vi "ORS_Fit_Recalibration_Fringes_Jay.vi"(0 "polynomial order":i32=2, 1 "n Recalibration Fringes":dbl[][](array[numeric]), 5 "polynomial fit algorithm":T1(ring), 7 "moving average half width":i32=1, 9 "interpolation method":i32(ring)=2 items=["nearest", "linear", "spline", "cubic Hermite", "Lagrange"], 11 "doPolyFit":bool, 12 "Offset":i32, 14 "Length":i32) -> (4 "maxphase":dbl, 6 "phase":dbl[](array[numeric]) format="%0.2f", 10 "inverted phase":dbl[](array[numeric]) format="%0.2f", 15 "rel.phase error":dbl[](array[numeric]) format="%0.2f")   [LabVIEW 2024]
uses:
  <vilib>/Analysis/baseanly.llb/Mean (DBL).vi
  <vilib>/Analysis/3filter.llb/Zero Phase Filter (DBL).vi
  <vilib>/Analysis/NI_AALPro.lvlib
  <vilib>/ptbypt/NI_PtbyPt.lvlib
  <vilib>/Analysis/NI_AALBase.lvlib
panel:
  out "CaliBackgroud":dbl[](graph)
  out "size(s)":i32[](array[numeric])
  out "Input":dbl[][](graph)
  out "Waveform Graph":dbl[](graph)
  out "element":dbl
  out "Mean fringes":dbl[][](graph)
  out "Unwrapped Hilbert phase":dbl[][](graph)
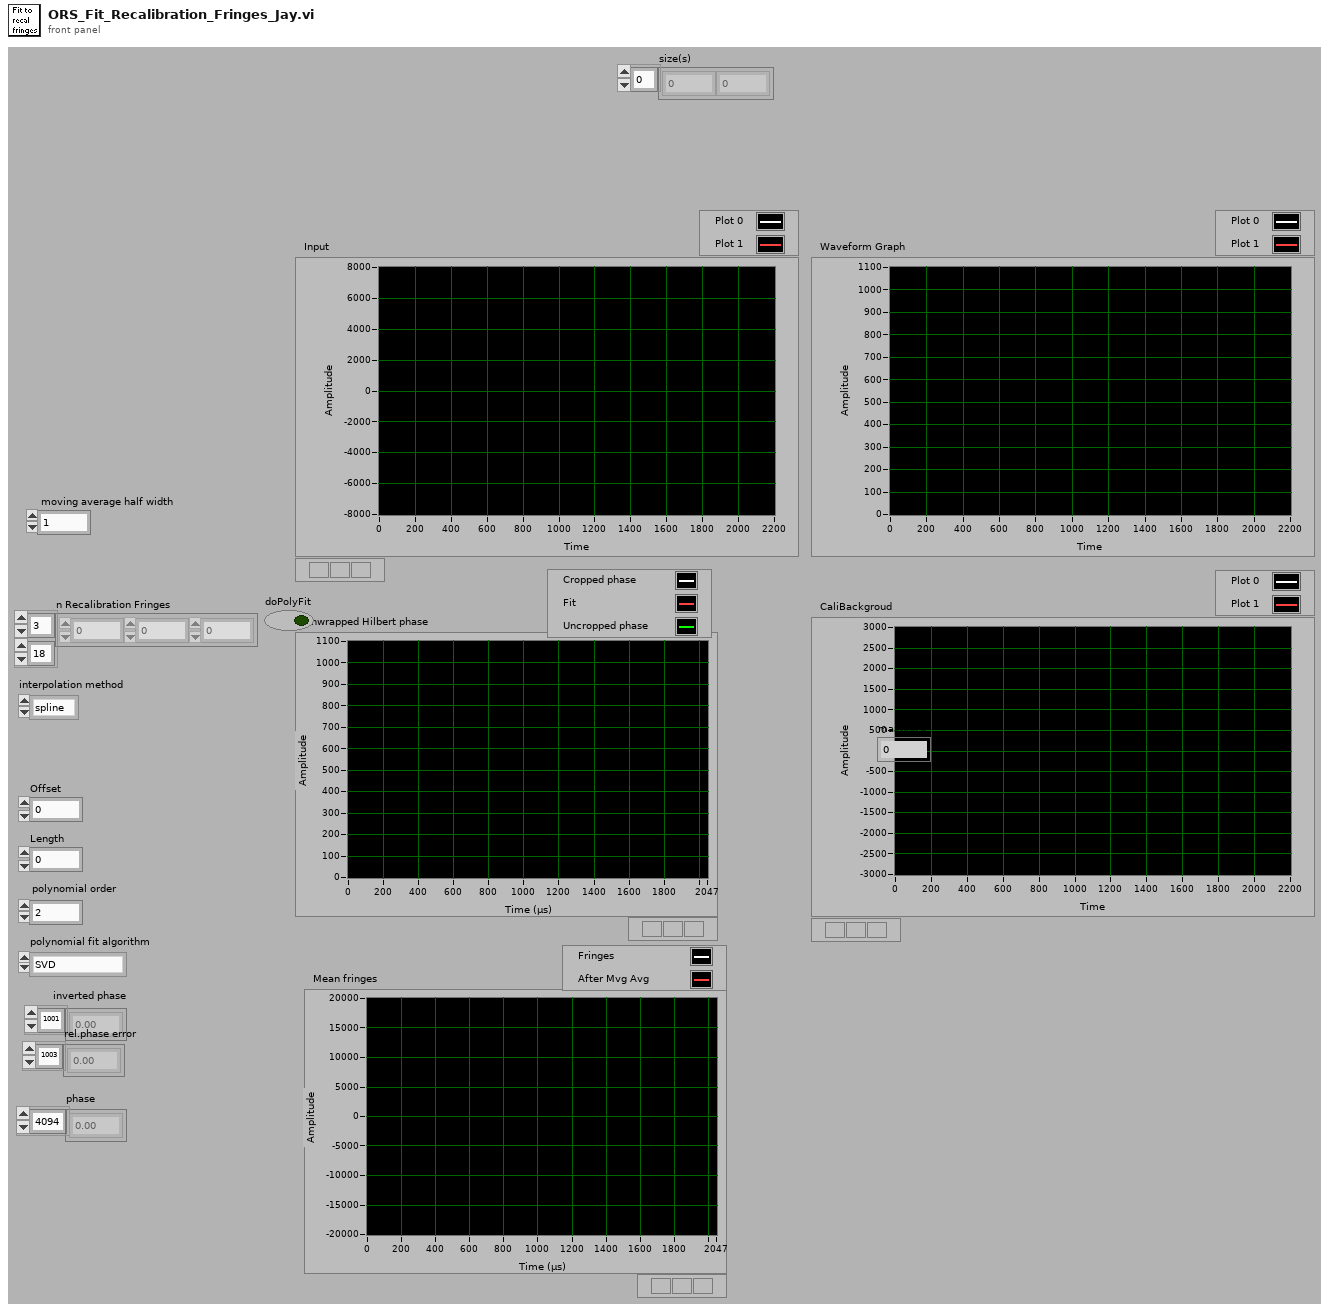
[diagram p1: front panel]
types:
  T1 = enum32{"SVD", "Givens", "Givens2", "Householder", "LU Decomposition", "Cholesky"}
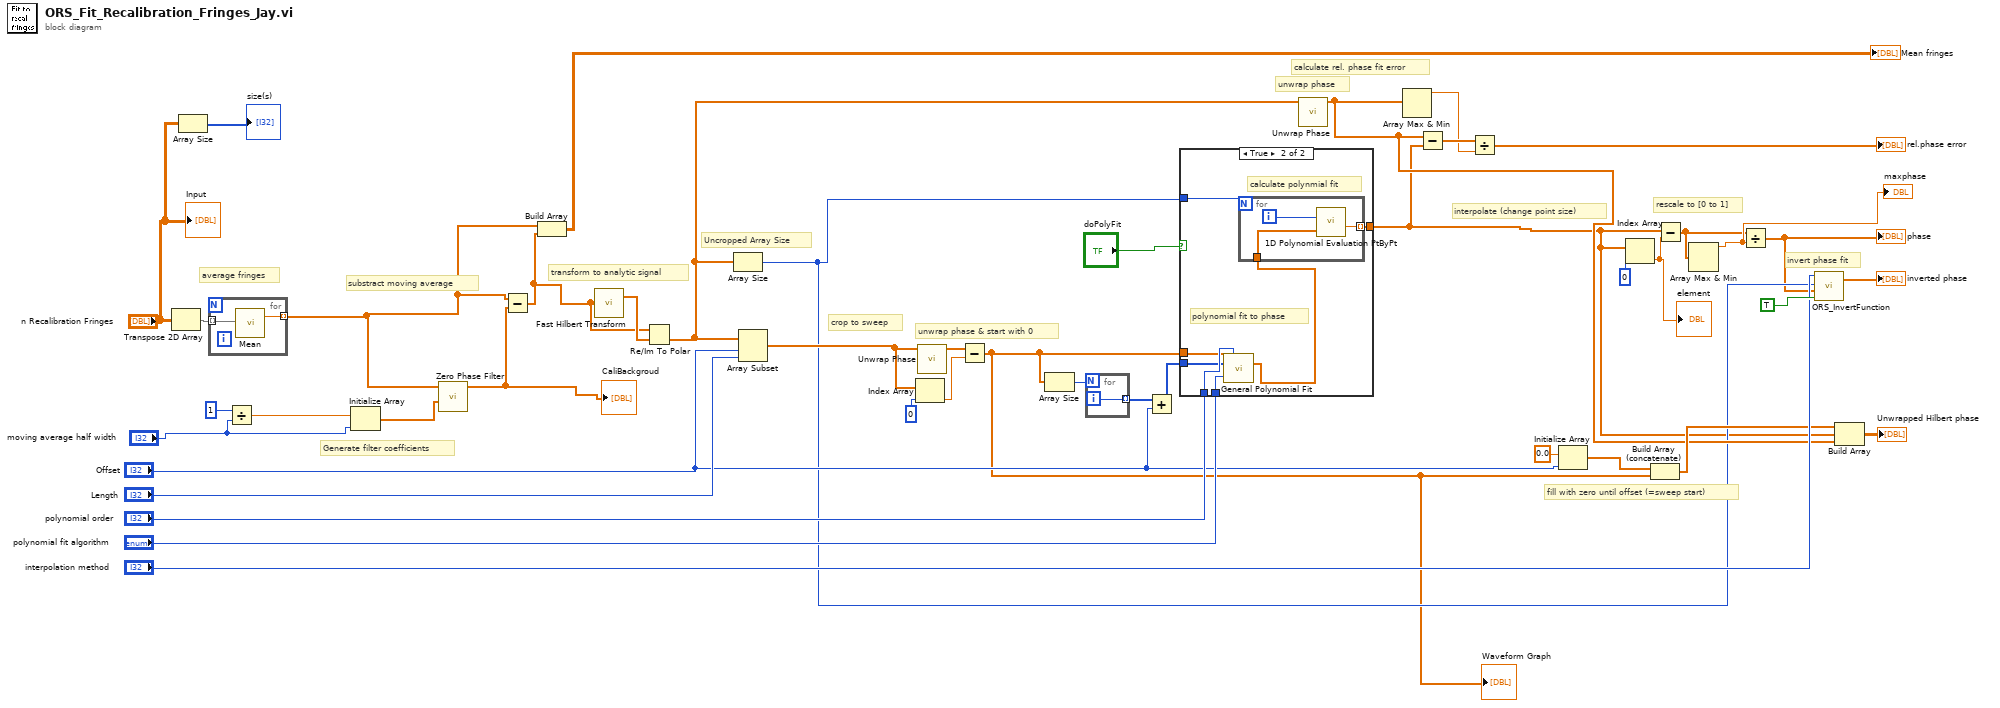
[diagram p0: block diagram]
diagram:
  # "Generate filter coefficients"
  # "transform to analytic signal"
  # "unwrap phase"
  # "average fringes"
  # "fill with zero until offset (=sweep start)"
  # "unwrap phase & start with 0"
  # "Uncropped Array Size"
  # "calculate rel. phase fit error"
  # "rescale to [0 to 1]"
  # "interpolate (change point size)"
  # "substract moving average"
  # "invert phase fit"
  # "crop to sweep"
  n1 = Transpose 2D Array(2D array="n Recalibration Fringes") -> (transposed array=w11:dbl[][])
  n2 = Array Size(array="n Recalibration Fringes") -> (size(s)=→"size(s)":i32[])
  n3 = for {
    tunnel: w11 -> [w46] mode=indexing
    tunnel: [w45] -> w10 mode=indexing
    n4 = call-poly <vilib>:"Mean.vi"("X"=w46) -> ("mean"=w45:dbl)  [unwired: 1 out]
  }
  n5 = Divide(x=1, y="moving average half width") -> (x/y=w3:dbl)
  n6 = Initialize Array(w3, "moving average half width") -> (w4:dbl[])
  n7 = call-poly <vilib>:"Zero Phase Filter.vi"("Forward Coefficients"=w4, "X"=w10) -> ("Filtered X"=w5:dbl[])  [unwired: 8 in, 1 out]
  "CaliBackgroud" <- w5
  n8 = Subtract(x=w10, y=w5) -> (x-y=w13:dbl[])
  n9 = Build Array(w10, w13) -> (→"Mean fringes":dbl[][])
  n10 = call <vilib>:"Fast Hilbert Transform.vi"("X"=w13) -> ("Hilbert{X}"=w23:dbl[])  [unwired: 1 out]
  n11 = Re/Im To Polar(2:w23, 3:w13) -> (0:w12:dbl[])  [unwired: 1 out]
  n12 = Array Size(array=w12) -> (size(s)=w19:i32)
  n13 = Array Subset(array=w12, index="Offset", length="Length") -> (w22:dbl[])
  n14 = Index Array(array=w22, index=0) -> (element=w28:dbl)
  n15 = call <vilib>:"Unwrap Phase.vi"("Phase"=w22) -> ("Unwrapped Phase"=w21:dbl[])  [unwired: 9 in, 1 out]
  n16 = Subtract(x=w21, y=w28) -> (x-y=w9:dbl[])
  "Waveform Graph" <- w9
  n17 = Array Size(array=w9) -> (size(s)=w39:i32)
  n18 = for {
    N: w39 -> [_]
    tunnel: [w47] -> w38 mode=indexing
    i -> [w47]
  }
  n19 = Add(x=w38, y="Offset") -> (x+y=w37:i32[])
  n20 = case shown="True" "doPolyFit" {
    tunnel: "polynomial fit algorithm" -> [_ w55]
    tunnel: "polynomial order" -> [_ w54]
    tunnel: w37 -> [_ w53]
    tunnel: w9 -> [w48 w52]
    tunnel: w19 -> [_ w51]
    tunnel: [w48 w49] -> w15
    frame False {
    }
    frame True {
      # "calculate polynmial fit"
      # "polynomial fit to phase"
      n21 = call <vilib>:"General Polynomial Fit.vi"("Y"=w52, "polynomial order"=w54, "X"=w53, "algorithm"=w55) -> ("Polynomial Coefficients"=w50:dbl[])  [unwired: 8 in, 3 out]
      n22 = for {
        N: w51 -> [_]
        tunnel: [w58] -> w49 mode=indexing
        tunnel: w50 -> [w56]
        i -> [w57]
        n23 = call <vilib>:"1D Polynomial Evaluation PtByPt.vi"("Coefficients: a"=w56, "x"=w57) -> ("y"=w58:dbl)
      }
    }
  }
  n24 = call <vilib>:"Unwrap Phase.vi"("Phase"=w12) -> ("Unwrapped Phase"=w26:dbl[])  [unwired: 9 in, 1 out]
  n25 = Array Max & Min(array=w26) -> (max value=w35:dbl)  [unwired: 3 out]
  n26 = Subtract(x=w26, y=w15) -> (x-y=w36:dbl[])
  n27 = Divide(x=w36, y=w35) -> (x/y=→"rel.phase error":dbl[])
  n28 = Initialize Array(0.0 ("element"), "Offset") -> (w33:dbl[])
  n29 = Index Array(array=w15, index=0 ("Index")) -> (element=w17:dbl)
  "element" <- w17
  n30 = Build Array (concatenate)(w33, w9) -> (w30:dbl[])
  n31 = Subtract(x=w15, y=w17) -> (x-y=w31:dbl[])
  n32 = Array Max & Min(array=w31) -> (max value=w41:dbl)  [unwired: 3 out]
  "maxphase" <- w41
  n33 = Divide(x=w31, y=w41) -> (x/y=w14:dbl[])
  "phase" <- w14
  n34 = call "ORS_InvertFunction.vi"("Rescale to input"=TRUE, "input"=w14, "number of points"=w19, "method"="interpolation method") -> ("inverted output"=→"inverted phase":dbl[])  [unwired: 1 in]
  n35 = Build Array(w30, w15, w26) -> (→"Unwrapped Hilbert phase":dbl[][])
  "Input" <- "n Recalibration Fringes"
